vi "XNET UDP Socket Open.vi"(6 "local interface":string, 7 "stack":refnum<k21>, 8 "error in":errorcluster, 11 "local port":u16) -> (0 "error out":errorcluster, 2 "actual local port":u16, 3 "socket":refnum<k20>)   [LabVIEW 2018]
doc: "Opens a UDP socket to send a datagram to a single receiver on the port you specify. If you want to send a single datagram to multiple receivers in parallel, use the XNET UDP Multicast Open node."
uses:
  nixlvapi.dll
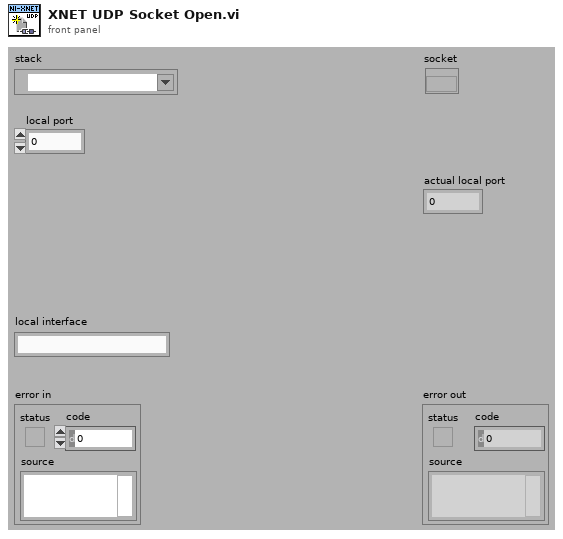
[diagram p1: front panel]
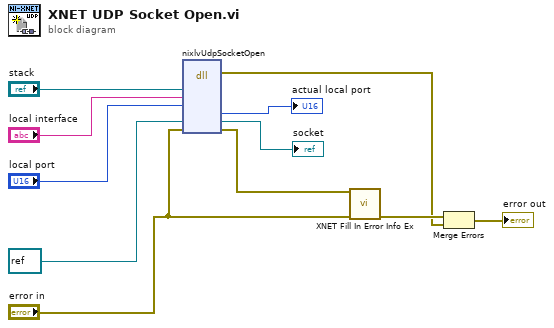
[diagram p0: block diagram]
diagram:
  n1 = dll-call lib="nixlvapi.*" fn="nixlvUdpSocketOpen" label="Call Library"("stackRef"="stack", "localInterface"="local interface", "localPort"="local port", "socketRefObjPtr"=refnum<k20> refnum ("socket"), "errorInOut"="error in") -> (error out=w9:errorcluster, "actualLocalPort"=→"actual local port":u16, "socketRefObjPtr"=→"socket":refnum<k20>, "errorInOut"=w11:errorcluster)  [unwired: 3 in, 6 out]
  n2 = call "XNET Fill In Error Info Ex.vi"("error xnet"=w11, "error in"="error in") -> ("error out"=w10:errorcluster)  [unwired: 13 in]
  n3 = Merge Errors(w10, w9) -> (→"error out":errorcluster)
